vi "JoyStickEvent.vi"(8 "error in":errorcluster, 10 "UserEvent_Handle":T1, 11 "device ID":refnum<k1>) -> ()   [LabVIEW 2013]
uses:
  Joystick_UserEvent.ctl
  ControlDef/QuitProg.vi
  <vilib>/Utility/inputDevices.llb/joystickAcquire.vi
panel:
  out "raw response":i32[](array[numeric])
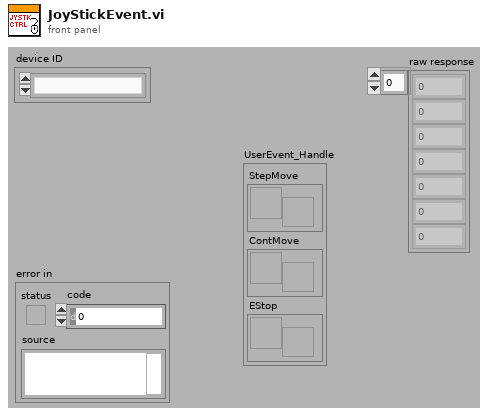
[diagram p1: front panel]
types:
  T1 = typedef "Joystick_UserEvent.ctl" = cluster{"StepMove":refnum<user-event>, "ContMove":refnum<user-event>, "EStop":refnum<user-event>}
  T2 = cluster{"X axis":i32, "Y axis":i32, "Z axis":i32, "X axis rotation":i32, "Y axis rotation":i32, "Z axis rotation":i32, "U axis":i32, "V axis":i32}
  T3 = cluster{"pov 1":i32, "pov 2":i32, "pov 3":i32, "pov 4":i32}
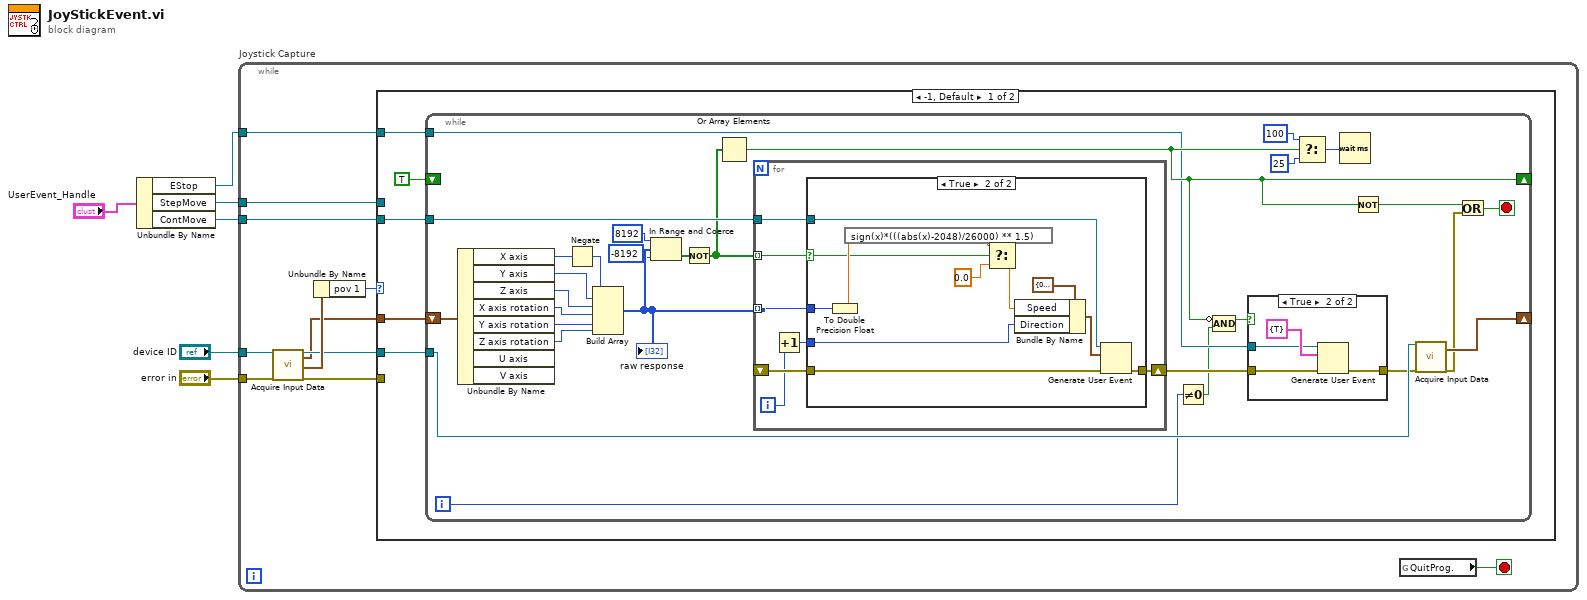
[diagram p0: block diagram]
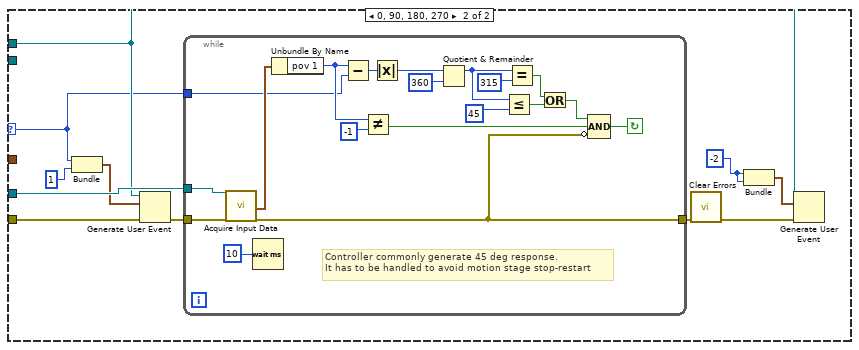
[diagram p4: hidden frame]
diagram:
  n1 = Unbundle By Name("UserEvent_Handle") -> ("EStop"=w1:refnum<user-event>, "StepMove"=w3:refnum<user-event>, "ContMove"=w2:refnum<user-event>)
  n2 = while "Joystick Capture" {
    tunnel: "error in" -> [w16]
    tunnel: "device ID" -> [w17]
    tunnel: w3 -> [w15]
    tunnel: w2 -> [w8]
    tunnel: w1 -> [w7]
    stop <- w14 stop-if-true
    n3 = call-poly <vilib>:"Acquire Input Data.vi"("device ID"=w17, "error in (no error)"=w16) -> ("device ID"=w10:refnum<k1>, "axis info"=w9:T2, "direction info"=w13:T3, "error out"=w11:errorcluster)  [unwired: 13 in, 1 out]
    n4 = Unbundle By Name(w13) -> ("pov 1"=w12:i32)
    n5 = case shown="-1, Default" w12 {
      selector: w12 -> [_ w80]
      tunnel: w11 -> [_ w85]
      tunnel: w10 -> [w20 w87]
      tunnel: w15 -> [_ w83]
      tunnel: w9 -> [w22 _]
      tunnel: w8 -> [w21 _]
      tunnel: w7 -> [w18 _]
      frame -1, Default {
        n6 = while {
          tunnel: w21 -> [w47]
          tunnel: w20 -> [w46]
          shift-right: [w45] -> _
          shift-left: w22 -> [w51]
          shift-right: [w32] -> _
          shift-left: TRUE -> [_]
          tunnel: w18 -> [w29]
          i -> [w24]
          stop <- w31 stop-if-true
          n7 = Unbundle By Name(w51) -> ("X axis"=w50:i32, "Y axis"=w49:i32, "Z axis"=w48:i32, "X axis rotation"=w44:i32, "Y axis rotation"=w43:i32, "Z axis rotation"=w42:i32)  [unwired: 2 out]
          n8 = Negate(x=w50) -> (-x=w23:i32)
          n9 = Build Array(w23, w49, w48, w44, w43, w42) -> (w41:i32[])
          "raw response" <- w41
          n10 = In Range and Coerce(upper limit=8192, x=w41, lower limit=-8192) -> (In Range?=w38:bool[])  [unwired: 1 out]
          n11 = Not(x=w38) -> (.not. x?=w27:bool[])
          n12 = Or Array Elements(Boolean array=w27) -> (logical OR=w32:bool)
          n13 = for {
            tunnel: w41 -> [w63] mode=indexing
            tunnel: w47 -> [w62]
            shift-right: [w61] -> w37
            shift-left: _ -> [w59]
            tunnel: w27 -> [w60] mode=indexing
            i -> [w57]
            n14 = Increment(x=w57) -> (x+1=w58:i32)
            n15 = case shown="True" w60 {
              selector: w60 -> [_ w65]
              tunnel: w63 -> [_ w76]
              tunnel: w62 -> [_ w75]
              tunnel: [w64 w72] -> w61
              tunnel: w59 -> [w64 w67]
              tunnel: w58 -> [_ w66]
              frame False {
              }
              frame True {
                n16 = To Double Precision Float(number=w76) -> (double precision float=w73:dbl)
                n17 = expression code="sign(x)*(((abs(x)-2048)/26000) ** 1.5)"(w73) -> (w74:dbl)
                n18 = Select(t=w74, s=w65, f=0.0 ("t")) -> (s? t:f=w69:dbl)
                n19 = Bundle By Name(cluster=cluster{"Direction":i32, "Speed":dbl} {"Direction"=0, "Speed"=0.0} ("event data"), "Speed"=w69, "Direction"=w66) -> (w70:cluster{"Direction":i32, "Speed":dbl})
                n20 = Generate User Event(user event=w75, event data cluster=w70, error in=w67) -> (error out=w72:errorcluster)  [unwired: 1 in, 1 out]
              }
            }
          }
          n21 = Not Equal To 0?(x=w24) -> (x != 0?=w25:bool)
          n22 = Compound Arithmetic op=AND(invert w32, w25) -> (w26:bool)
          n23 = case shown="True" w26 {
            tunnel: w37 -> [w52 w55]
            tunnel: [w52 w54] -> w30
            tunnel: w29 -> [_ w53]
            frame False {
            }
            frame True {
              n24 = Generate User Event(user event=w53, event data cluster=cluster{bool} {TRUE} ("event data"), error in=w55) -> (error out=w54:errorcluster)  [unwired: 1 in, 1 out]
            }
          }
          n25 = Select(t=u32 100 ("millisecond timer value"), s=w32, f=u32 25 ("millisecond timer value")) -> (s? t:f=w33:u32)
          n26 = Wait (ms)(milliseconds to wait=w33) -> ()  [unwired: 1 out]
          n27 = Not(x=w32) -> (.not. x?=w36:bool)
          n28 = call-poly <vilib>:"Acquire Input Data.vi"("device ID"=w46, "error in (no error)"=w30) -> ("axis info"=w45:T2, "error out"=w28:errorcluster)  [unwired: 13 in, 3 out]
          n29 = Or(x=w36, y=w28) -> (x .or. y?=w31:bool)
        }
      }
      frame 0, 90, 180, 270 {
        w78 = -2 ("event data")
        n30 = Bundle("pov 1"=w80, 1) -> (w81:cluster{"pov 1":i32, i32})  [unwired: 1 in]
        n31 = Generate User Event(user event=w83, event data cluster=w81, error in=w85) -> (error out=w86:errorcluster)  [unwired: 1 in, 1 out]
        n32 = while {
          tunnel: w86 -> [w105]
          tunnel: w87 -> [w104]
          tunnel: [w88] -> w84
          tunnel: w80 -> [w95]
          stop <- w97 continue-if-true
          # "Controller commonly generate 45 deg response.\nIt has to be handled to avoid motion stage stop-restart"
          n33 = call-poly <vilib>:"Acquire Input Data.vi"("device ID"=w104, "error in (no error)"=w105) -> ("direction info"=w103:T3, "error out"=w88:errorcluster)  [unwired: 13 in, 3 out]
          n34 = Wait (ms)(milliseconds to wait=u32 10) -> ()  [unwired: 1 out]
          n35 = Unbundle By Name(w103) -> ("pov 1"=w101:i32)
          n36 = Subtract(x=w101, y=w95) -> (x-y=w100:i32)
          n37 = Not Equal?(x=w101, y=-1) -> (x != y?=w98:bool)
          n38 = Absolute Value(x=w100) -> (abs(x)=w96:i32)
          n39 = Quotient & Remainder(x=w96, y=360) -> (x-y*floor(x/y)=w92:i32)  [unwired: 1 out]
          n40 = Less Or Equal?(x=w92, y=45) -> (x <= y?=w90:bool)
          n41 = Equal?(x=w92, y=315) -> (x = y?=w91:bool)
          n42 = Or(x=w91, y=w90) -> (x .or. y?=w89:bool)
          n43 = Compound Arithmetic op=AND(w89, w98, invert w88) -> (w97:bool)
        }
        n44 = call <vilib>:"Clear Errors.vi"("error in (no error)"=w84) -> ("error out"=w82:errorcluster)  [unwired: 6 in]
        n45 = Bundle("event data"=w78, "event data"=w78) -> (w77:cluster{"event data":i32, "event data":i32})  [unwired: 1 in]
        n46 = Generate User Event(user event=w83, event data cluster=w77, error in=w82) -> ()  [unwired: 1 in, 2 out]
      }
    }
    n47 = global read "QuitProg.vi" "QuitProg."() -> (w14:bool)
  }
